vi "Set State.vi"(8 "error in (no error)":errorcluster, 10 "State":T1, 11 "Car Wash Controller in":refnum<class "Car Wash Controller.lvclass">) -> (0 "error out":errorcluster, 3 "Car Wash Controller out":refnum<class "Car Wash Controller.lvclass">)   [LabVIEW 2019, in "Car Wash Controller.lvlib" / "Car Wash Controller.lvclass"]
uses:
  Car Wash Controller.lvclass
  States -Enum.ctl
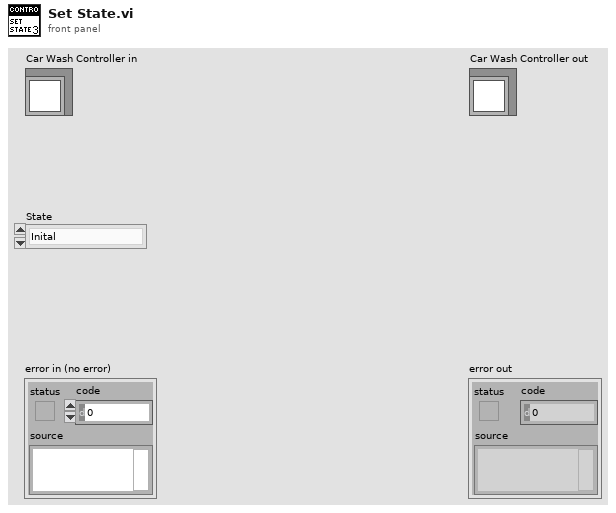
[diagram p1: front panel]
types:
  T1 = typedef "Car Wash Controller.lvlib/Car Wash Controller.lvclass/States -Enum.ctl" = enum16{"Inital", "Wait for Start", "Start", "Wait for Vehicle Position", "Wash Step Execution", "Wash Step/Cycle Completion", "Wash Exit", "Wash Abort/Terminate State"}
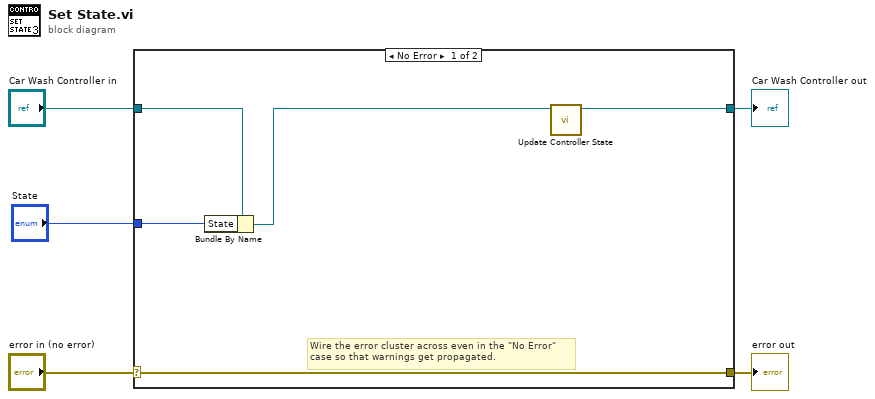
[diagram p0: block diagram]
diagram:
  n1 = case shown="No Error" "error in (no error)" {
    selector: "error in (no error)" -> [w10 w12]
    tunnel: [w10 w12] -> w4
    tunnel: [w7 w11] -> w2
    tunnel: "Car Wash Controller in" -> [w8 w11]
    tunnel: "State" -> [w9 _]
    frame No Error {
      # "Wire the error cluster across even in the \"No Error\"\ncase so that warnings get propagated."
      n2 = Bundle By Name(cluster=w8, "State"=w9) -> (w6:refnum<class "Car Wash Controller.lvclass">)
      n3 = call "Update Controller State.vi"("Car Wash Controller in"=w6) -> ("Car Wash Controller out"=w7:refnum<class "Car Wash Controller.lvclass">)  [unwired: 9 in, 1 out]
    }
    frame Error {
    }
  }
  "error out" <- w4
  "Car Wash Controller out" <- w2
